vi "ReadAndSaveData.vi"(0 "object in":refnum<class "CetoniPump.lvclass">, 1 "tdms file":refnum<k34>, 2 "group name in (Untitled)":string, 5 "error in (no error)":errorcluster) -> (14 "object out":refnum<class "CetoniPump.lvclass">, 19 "error out":errorcluster)   [LabVIEW 2023, in "CetoniPump.lvclass"]
uses:
  CetoniPump.lvclass
  CetoniPump.lvclass/CetoniPump.ctl
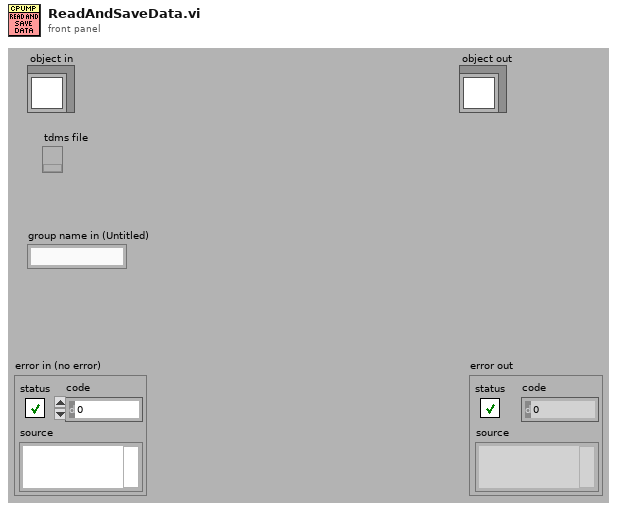
[diagram p1: front panel]
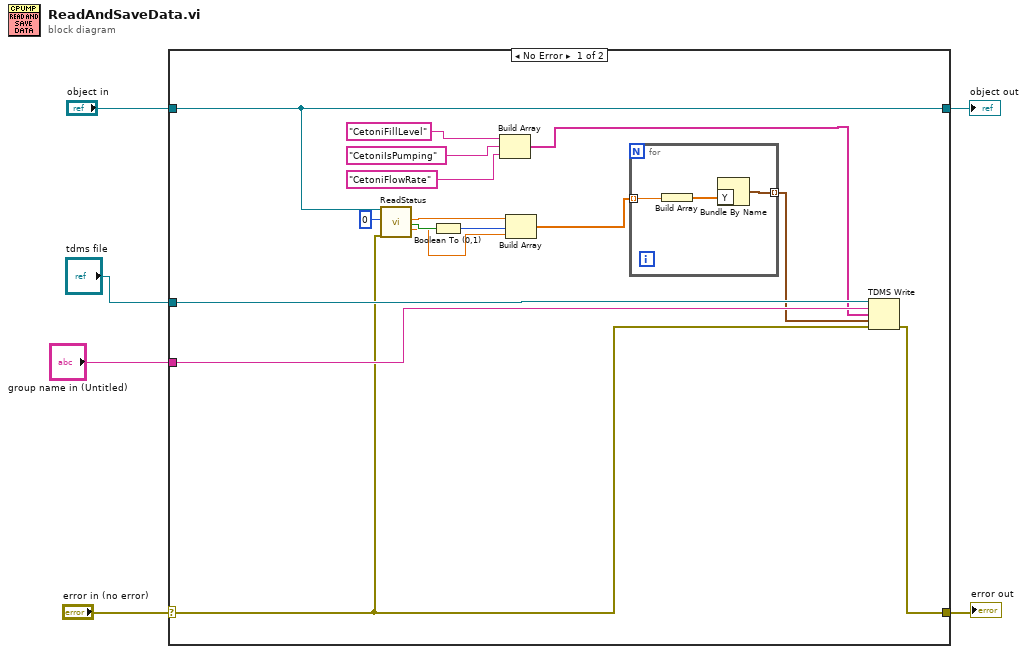
[diagram p0: block diagram]
diagram:
  n1 = case shown="No Error" "error in (no error)" {
    selector: "error in (no error)" -> [w18 w27]
    tunnel: [w17 w27] -> w5
    tunnel: [w22 w26] -> w3
    tunnel: "object in" -> [w22 w26]
    tunnel: "tdms file" -> [w20 _]
    tunnel: "group name in (Untitled)" -> [w19 _]
    frame No Error {
      n2 = call-dynamic "ReadStatus.vi"("object in"=w22, "index"=0, "error in (no error)"=w18) -> ("Fill Level"=w16:dbl, "Is pumping"=w15:bool, "Actual Flow Rate"=w13:dbl)  [unwired: 12 in, 2 out]
      n3 = Boolean To (0,1)(Boolean=w15) -> (0, 1=w14:i16)
      n4 = Build Array("CetoniFillLevel", "CetoniIsPumping", "CetoniFlowRate") -> (w7:string[])
      n5 = Build Array(w16, w14, w13) -> (w9:dbl[])
      n6 = for {
        tunnel: w9 -> [w25] mode=indexing
        tunnel: [w23] -> w8 mode=indexing
        n7 = Build Array(w25) -> (w24:dbl[])
        n8 = Bundle By Name("Y"=w24) -> (w23:waveform(dbl))  [unwired: 1 in]
      }
      n9 = TDMS Write(0:w20, 5:w19, 7:w7, 9:w8, 11:w18) -> (15:w17:errorcluster)  [unwired: 1 in, 3 out]
    }
    frame Error {
    }
  }
  "error out" <- w5
  "object out" <- w3
